vi "Teleop Cmd Send co-pilot.vi"(6 "Co_fifo":refnum<k33>, 7 "Epsilon":dbl, 8 "error in (no error)":errorcluster, 10 "mechanism log":refnum<file>, 11 "Co-Pilot Data":T1) -> (0 "error out":errorcluster)   [LabVIEW 2014]
uses:
  Co-Pilot_game_control.ctl
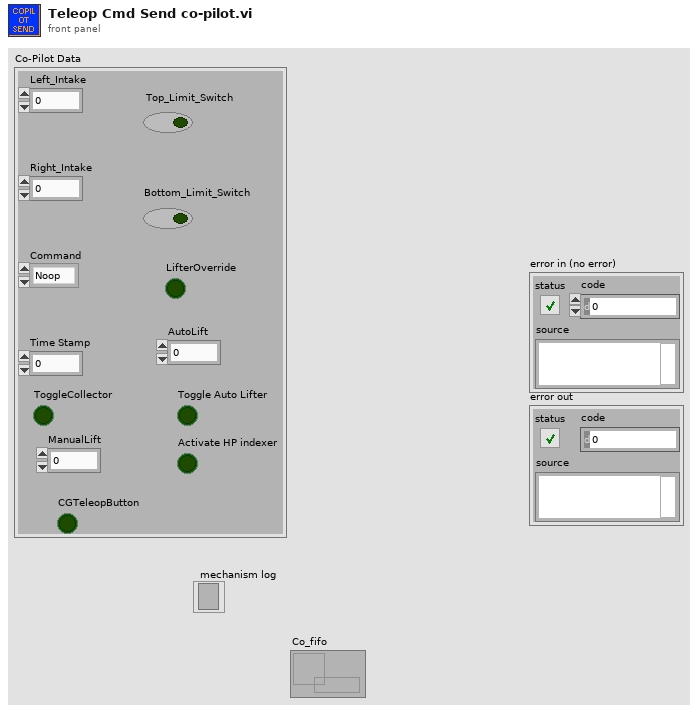
[diagram p1: front panel]
types:
  T1 = typedef "Co-Pilot_game_control.ctl" = cluster{"Left_Intake":dbl, "Right_Intake":dbl, "Time Stamp":u32, "Command":enum16{"Noop", "Flagged"}, "ToggleCollector":bool, "ManualLift":dbl, "Top_Limit_Switch":bool, "Bottom_Limit_Switch ":bool, "LifterOverride":bool, "AutoLift":i32, "Toggle Auto Lifter":bool, "Activate HP indexer":bool, "CGTeleopButton":bool}
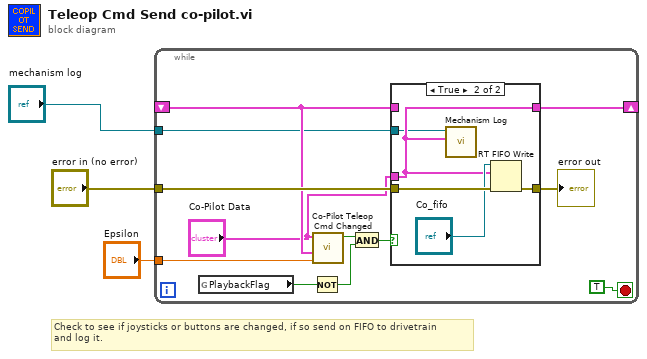
[diagram p0: block diagram]
diagram:
  # "Check to see if joysticks or buttons are changed, if so send on FIFO to drivetrain\nand log it."
  n1 = while "Prev Right\nPrev Right Value" {
    tunnel: "error in (no error)" -> [w14]
    tunnel: "Epsilon" -> [w13]
    shift-right: [w12] -> _
    shift-left: _ -> [w11]
    tunnel: "mechanism log" -> [w4]
    stop <- TRUE stop-if-true
    n2 = global read "PlaybackOn" "PlaybackFlag"() -> (w8:bool)
    n3 = Not(x=w8) -> (.not. x?=w9:bool)
    n4 = call "Co-Pilot Teleop Cmd Changed.vi"("New_Co-Pilot Data"="Co-Pilot Data", "Co-Pilot Data"=w11, "Epsilon"=w13) -> ("Boolean"=w10:bool)  [unwired: 6 in]
    n5 = And(x=w10, y=w9) -> (x .and. y?=w7:bool)
    n6 = case shown="True" w7 {
      tunnel: [w17 w22] -> w6
      tunnel: w14 -> [w17 w21]
      tunnel: "Co-Pilot Data" -> [_ w19]
      tunnel: [w16 w19] -> w12
      tunnel: w11 -> [w16 _]
      tunnel: w4 -> [_ w18]
      frame False {
      }
      frame True {
        n7 = call "Mechanism Log.vi"("Co-Pilot Data in"=w19, "Byte Stream File in"=w18) -> ()  [unwired: 10 in]
        n8 = RT FIFO Write(0:"Co_fifo", 1:w19, 3:w21) -> (11:w22:errorcluster)  [unwired: 2 in, 3 out]
      }
    }
    "error out" <- w6
  }
